vi "LVClass_Camera get Internal image.vi"(0 "Camera in":refnum<class "Camera.lvclass">, 11 "error in (no error)":errorcluster) -> (4 "Camera out":refnum<class "Camera.lvclass">, 6 "remove background?":bool, 15 "error out":errorcluster)   [LabVIEW 2020, in "Camera.lvclass"]
doc: "Retrieve last captured image. see Imop_Camera_AsyncImageReady.\n\n<B>CameraIn</B> : Camera object.\n<B>CameraOut</B> : Camera object.\n<B>remove_background</B> : Boolean which indicates if background is substracted.\n\nRetrieve last captured image. see Imop_Camera_AsyncImageReady.\n\nCaptured image with or without any post-processing applied have been updated into the camera object. To get those image object to use, please use LVClass_Camera Read Image.vi or LVClass_Camera Read RAW Image.vi method"
uses:
  Camera.lvclass
  Camera.lvclass/Camera.ctl
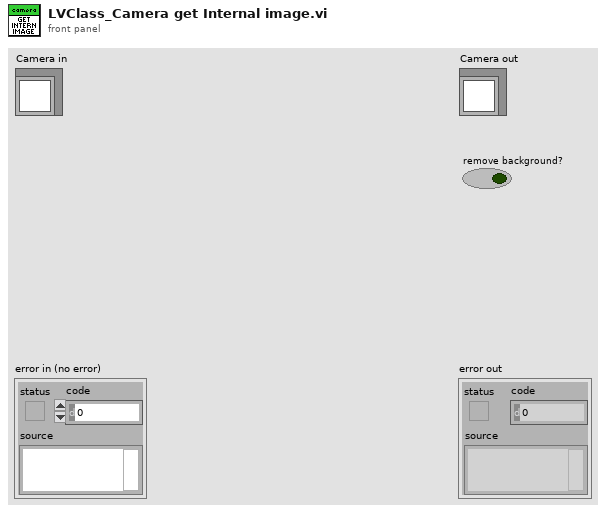
[diagram p1: front panel]
types:
  T1 = typedef "CameraAcquisitionState.ctl" = enum16{"Stop", "Live"}
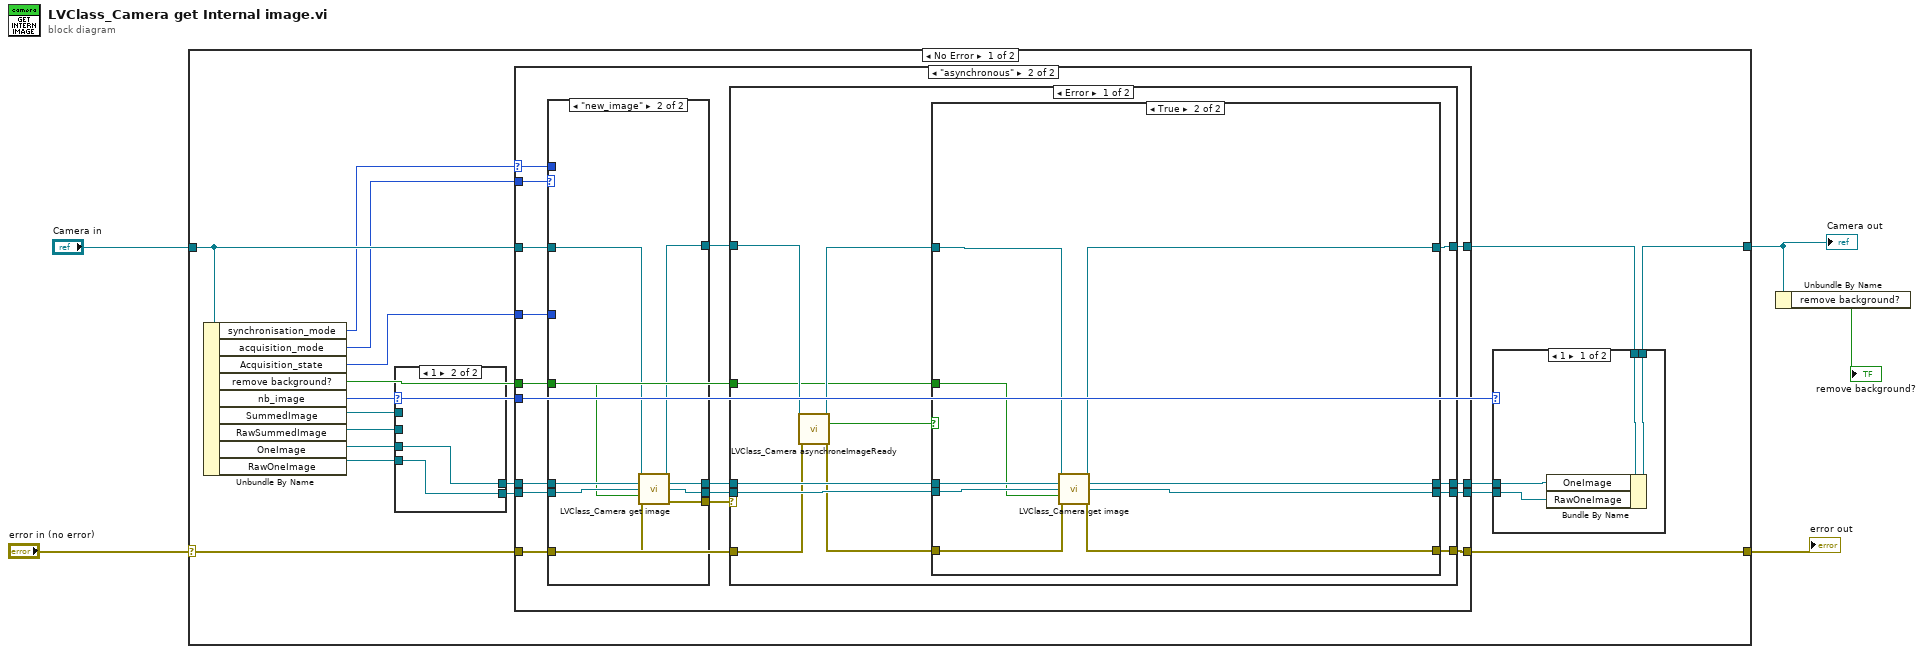
[diagram p0: block diagram]
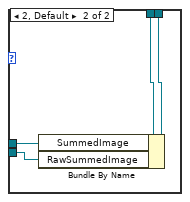
[diagram p2: hidden frame]
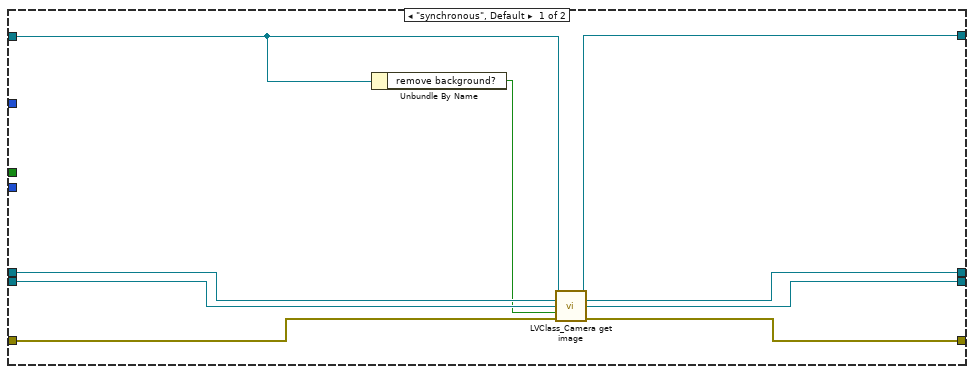
[diagram p4: hidden frame]
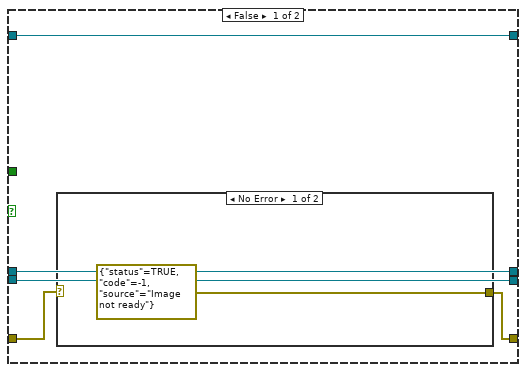
[diagram p5: hidden frame]
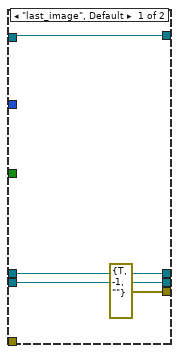
[diagram p8: hidden frame]
diagram:
  n1 = case shown="No Error" "error in (no error)" {
    selector: "error in (no error)" -> [w18 w107]
    tunnel: [w17 w107] -> w1
    tunnel: [w8 w106] -> w4
    tunnel: "Camera in" -> [w16 w106]
    frame No Error {
      n2 = Unbundle By Name(w16) -> ("synchronisation_mode"=w13:enum16{"synchronous", "asynchronous"}, "acquisition_mode"=w15:enum16{"last_image", "new_image"}, "Acquisition_state"=w14:T1, "remove background?"=w6:bool, "nb_image"=w12:u32, "SummedImage"=w21:refnum<class "Image.lvclass">, "RawSummedImage"=w20:refnum<class "Image.lvclass">, "OneImage"=w19:refnum<class "Image.lvclass">, "RawOneImage"=w7:refnum<class "Image.lvclass">)
      n3 = case shown="1" w12 {
        tunnel: [w33 w35] -> w22
        tunnel: w20 -> [w32 _]
        tunnel: w21 -> [w33 _]
        tunnel: [w32 w34] -> w23
        tunnel: w19 -> [_ w35]
        tunnel: w7 -> [_ w34]
        frame 2, Default {
        }
        frame 1 {
        }
      }
      n4 = case shown="\"asynchronous\"" w13 {
        selector: w13 -> [_ w49]
        tunnel: w18 -> [w42 w55]
        tunnel: w16 -> [w39 w58]
        tunnel: [w44 w60] -> w9
        tunnel: [w43 w59] -> w17
        tunnel: w22 -> [w41 w52]
        tunnel: w23 -> [w40 w56]
        tunnel: w15 -> [_ w51]
        tunnel: w14 -> [_ w50]
        tunnel: w12 -> [_ _]
        tunnel: [w37 w47] -> w11
        tunnel: [w36 w46] -> w10
        tunnel: w6 -> [_ w45]
        frame "synchronous", Default {
          n5 = Unbundle By Name(w39) -> ("remove background?"=w38:bool)
          n6 = call "LVClass_Camera get image.vi"("Camera in"=w39, "Image"=w41, "Image RAW"=w40, "remove_background"=w38, "error in (no error)"=w42) -> ("Camera out"=w44:refnum<class "Camera.lvclass">, "Image (dup)"=w37:refnum<class "Image.lvclass">, "Image (dup) RAW"=w36:refnum<class "Image.lvclass">, "error out"=w43:errorcluster)  [unwired: 7 in]
        }
        frame "asynchronous" {
          n7 = case shown="\"new_image\"" w51 {
            tunnel: w58 -> [w96 w100]
            tunnel: [w96 w105] -> w57
            tunnel: w52 -> [w95 w104]
            tunnel: w56 -> [w94 w103]
            tunnel: w55 -> [_ w99]
            tunnel: [w94 w98] -> w54
            tunnel: [w95 w102] -> w53
            tunnel: w50 -> [_ _]
            tunnel: w49 -> [_ _]
            tunnel: [errorcluster {"status"=TRUE, "code"=-1, "source"=""} ("error out") w101] -> w48
            tunnel: w45 -> [_ w97]
            frame "last_image", Default {
            }
            frame "new_image" {
              n8 = call "LVClass_Camera get image.vi"("Camera in"=w100, "Image"=w104, "Image RAW"=w103, "remove_background"=w97, "error in (no error)"=w99) -> ("Camera out"=w105:refnum<class "Camera.lvclass">, "Image (dup)"=w102:refnum<class "Image.lvclass">, "Image (dup) RAW"=w98:refnum<class "Image.lvclass">, "error out"=w101:errorcluster)  [unwired: 7 in]
            }
          }
          n9 = case shown="Error" w48 {
            selector: w48 -> [_ w92]
            tunnel: [w72 w91] -> w60
            tunnel: [w71 w92] -> w59
            tunnel: w57 -> [w68 w91]
            tunnel: w55 -> [w62 _]
            tunnel: w54 -> [w67 w89]
            tunnel: w53 -> [w66 w90]
            tunnel: [w65 w90] -> w47
            tunnel: [w64 w89] -> w46
            tunnel: w45 -> [w63 _]
            frame Error {
              n10 = call "LVClass_Camera asynchroneImageReady.vi"("Camera in"=w68, "error in (no error)"=w62) -> ("Camera out"=w69:refnum<class "Camera.lvclass">, "ready"=w70:bool, "error out"=w61:errorcluster)  [unwired: 11 in]
              n11 = case shown="True" w70 {
                tunnel: [w77 w85] -> w72
                tunnel: [w76 w80] -> w71
                tunnel: w66 -> [w74 w88]
                tunnel: w67 -> [w73 w87]
                tunnel: w69 -> [w77 w86]
                tunnel: w61 -> [w75 w81]
                tunnel: [w74 w84] -> w65
                tunnel: [w73 w83] -> w64
                tunnel: w63 -> [_ w82]
                frame False {
                  n12 = case shown="No Error" w75 {
                    selector: w75 -> [_ w79]
                    tunnel: [errorcluster {"status"=TRUE, "code"=-1, "source"="Image not ready"} ("error out") w79] -> w76
                    frame No Error {
                    }
                    frame Error {
                    }
                  }
                }
                frame True {
                  n13 = call "LVClass_Camera get image.vi"("Camera in"=w86, "Image"=w88, "Image RAW"=w87, "remove_background"=w82, "error in (no error)"=w81) -> ("Camera out"=w85:refnum<class "Camera.lvclass">, "Image (dup)"=w84:refnum<class "Image.lvclass">, "Image (dup) RAW"=w83:refnum<class "Image.lvclass">, "error out"=w80:errorcluster)  [unwired: 7 in]
                }
              }
            }
            frame No Error {
            }
          }
        }
      }
      n14 = case shown="1" w12 {
        tunnel: w11 -> [w27 w31]
        tunnel: w10 -> [w26 w30]
        tunnel: w9 -> [w25 w29]
        tunnel: [w24 w28] -> w8
        frame 1 {
          n15 = Bundle By Name(cluster=w25, "OneImage"=w27, "RawOneImage"=w26) -> (w24:refnum<class "Camera.lvclass">)
        }
        frame 2, Default {
          n16 = Bundle By Name(cluster=w29, "SummedImage"=w31, "RawSummedImage"=w30) -> (w28:refnum<class "Camera.lvclass">)
        }
      }
    }
    frame Error {
    }
  }
  "error out" <- w1
  "Camera out" <- w4
  n17 = Unbundle By Name(w4) -> ("remove background?"=→"remove background?":bool)
